vi "DAQ_Assistant.vi"(1 "data":bool[](array[boolean]), 2 "Lines":string[](array[string]), 3 "data 2":bool, 4 "timeout (s)":dbl=10.0 format="%0.2f", 5 "error in":errorcluster, 7 "stop (T)":bool=TRUE) -> (14 "task out":refnum<k21>, 19 "error out":errorcluster)   [LabVIEW 2017]
doc: "Creates, edits, and runs tasks using NI-DAQmx. Refer to the NI-DAQmx Readme for a complete listing of devices NI-DAQmx supports.\n\nWhen you place this Express VI on the block diagram, the DAQ Assistant launches to create a new task. After you create a task, you can double-click the DAQ Assistant Express VI to edit that task. For continuous measurement or generation, place a while loop around the DAQ Assistant Express VI."
uses:
  <vilib>/DAQmx/write.llb/DAQmx Write.vi
  <vilib>/DAQmx/write.llb/DAQmx Write (Digital Bool 1Line 1Point).vi
  <vilib>/DAQmx/miscellaneous.llb/DAQmx Fill In Error Info.vi
  <vilib>/DAQmx/create/channels.llb/DAQmx Create Channel (DO-Digital Output).vi
  <resource>/objmgr/daqmx.rc
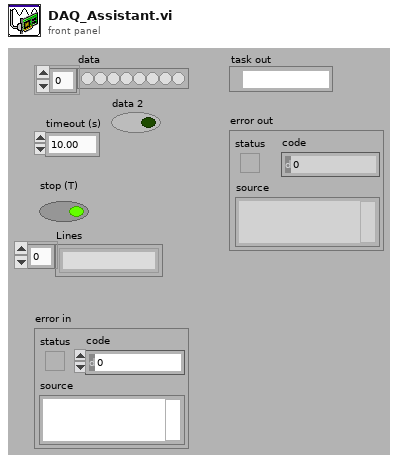
[diagram p1: front panel]
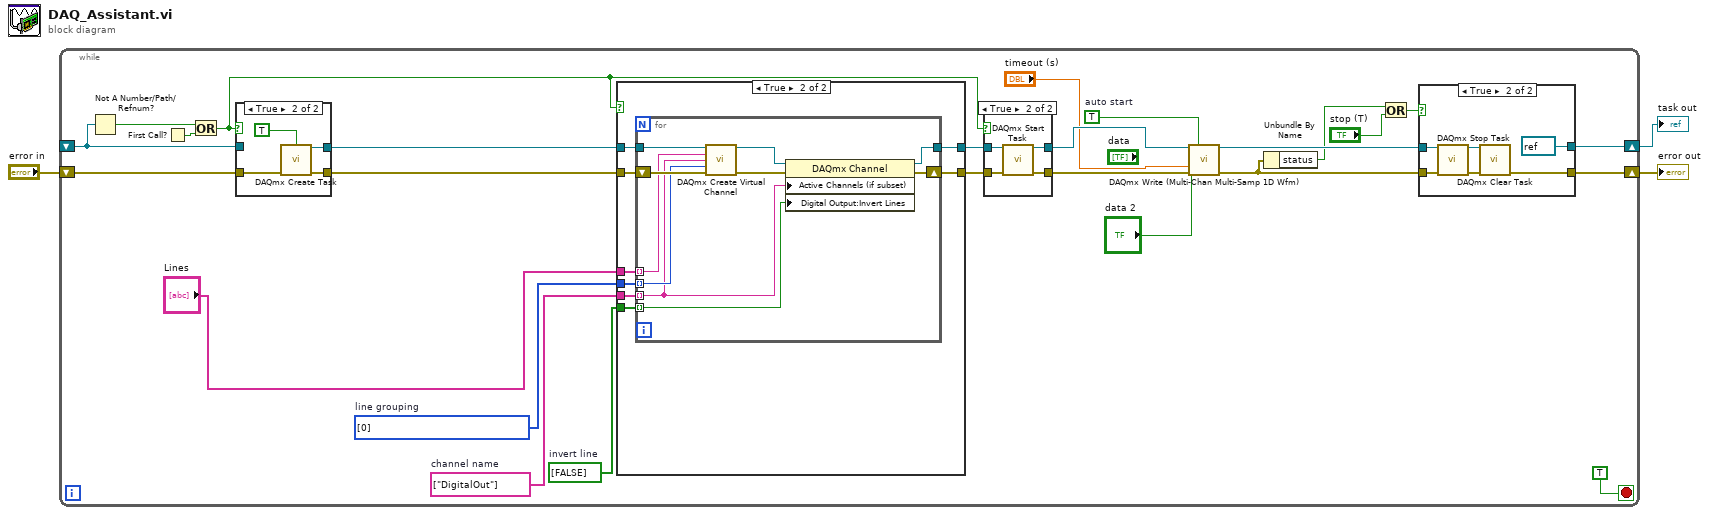
[diagram p0: block diagram]
diagram:
  n1 = while {
    shift-right: [w12] -> w1
    shift-left: _ -> [w26]
    shift-right: [w10] -> w2
    shift-left: "error in" -> [w27]
    stop <- TRUE stop-if-true
    w14 = TRUE  # auto start
    w20 = bool[] [FALSE]  # invert line
    w21 = i32[] [0] items=["one channel for each line", "one channel for all lines"]  # line grouping
    w22 = string[] ["DigitalOut"]  # channel name
    n2 = Not A Number/Path/Refnum?(number/path/refnum=w26) -> (NaN/Path/Refnum?=w25:bool)
    n3 = First Call?() -> (First Call?: T/F=w28:bool)
    n4 = Or(x=w25, y=w28) -> (x .or. y?=w19:bool)
    n5 = case shown="True" w19 {
      tunnel: [w65 w69] -> w24
      tunnel: w26 -> [w65 _]
      tunnel: [w64 w68] -> w23
      tunnel: w27 -> [w64 w66]
      frame False {
      }
      frame True {
        n6 = call <vilib>:"DAQmx Create Task.vi"("auto cleanup"=TRUE, "error in"=w66) -> ("task out"=w69:refnum<k21>, "error out"=w68:errorcluster)  [unwired: 12 in]
      }
    }
    n7 = case shown="True" w19 {
      tunnel: [w45 w46] -> w18
      tunnel: w24 -> [w45 w53]
      tunnel: [w44 w51] -> w17
      tunnel: w23 -> [w44 w52]
      tunnel: "Lines" -> [_ w50]
      tunnel: w22 -> [_ w49]
      tunnel: w21 -> [_ w48]
      tunnel: w20 -> [_ w47]
      frame False {
      }
      frame True {
        n8 = for {
          tunnel: w53 -> [w61]
          tunnel: w50 -> [w58] mode=indexing
          tunnel: w49 -> [w56] mode=indexing
          tunnel: w48 -> [w57] mode=indexing
          tunnel: w47 -> [w55] mode=indexing
          shift-right: [w59] -> w51
          shift-left: w52 -> [w60]
          tunnel: [w54] -> w46
          n9 = call-poly <vilib>:"DAQmx Create Virtual Channel.vi"("task in"=w61, "lines"=w58, "name to assign"=w56, "line grouping"=w57, "error in"=w60) -> ("task out"=w62:refnum<k21>, "error out"=w63:errorcluster)  [unwired: 9 in]
          n10 = property class="DAQmx Channel"(reference=w62, error in=w63, "Active Channels (if subset)"=w56, "Digital Output:Invert Lines"=w55) -> (reference out=w54:refnum<k21>, error out=w59:errorcluster)
        }
      }
    }
    n11 = case shown="True" w19 {
      tunnel: [w39 w42] -> w16
      tunnel: w18 -> [w39 w43]
      tunnel: [w38 w40] -> w15
      tunnel: w17 -> [w38 w41]
      frame False {
      }
      frame True {
        n12 = call <vilib>:"DAQmx Start Task.vi"("task/channels in"=w43, "error in"=w41) -> ("task out"=w42:refnum<k21>, "error out"=w40:errorcluster)  [unwired: 12 in]
      }
    }
    n13 = call-poly "DAQmx Write (Multi-Chan Multi-Samp 1D Wfm).vi"("task/channels in"=w16, "auto start"=w14, "data"="data 2", "timeout"="timeout (s)", "error in"=w15) -> ("task out"=w11:refnum<k21>, "error out"=w9:errorcluster)  [unwired: 8 in, 1 out]
    n14 = Unbundle By Name(w9) -> ("status"=w8:bool)
    n15 = Or(x=w8, y="stop (T)") -> (x .or. y?=w6:bool)
    n16 = case shown="True" w6 {
      tunnel: [w31 refnum<k21> refnum ("task in")] -> w12
      tunnel: w11 -> [w31 w37]
      tunnel: [w30 w34] -> w10
      tunnel: w9 -> [w30 w36]
      frame False {
      }
      frame True {
        n17 = call <vilib>:"DAQmx Stop Task.vi"("task/channels in"=w37, "error in"=w36) -> ("task out"=w33:refnum<k21>, "error out"=w35:errorcluster)  [unwired: 12 in]
        n18 = call <vilib>:"DAQmx Clear Task.vi"("task in"=w33, "error in"=w35) -> ("error out"=w34:errorcluster)  [unwired: 13 in]
      }
    }
  }
  "error out" <- w2
  "task out" <- w1
